vi "close.vi"(8 "error in":errorcluster, 11 "TEC runtime in":refnum<class "TEC runtime.lvclass">) -> (0 "error out":errorcluster)   [LabVIEW 2013, in "TEC runtime.lvclass"]
doc: "Provides an interface for terminating a module instance. While this interface performs no operations, a child should close and deallocate any open references or memory."
uses:
  TEC runtime.lvclass
  TEC runtime.lvclass/TEC runtime.ctl
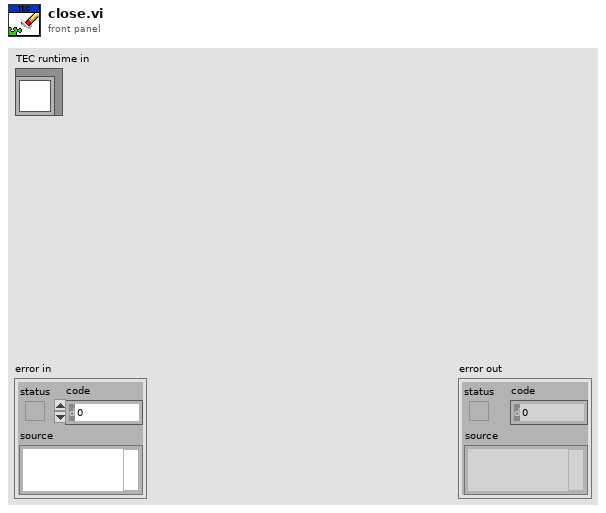
[diagram p1: front panel]
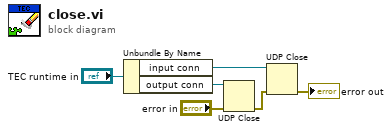
[diagram p0: block diagram]
diagram:
  n1 = Unbundle By Name("TEC runtime in") -> ("input conn"=w1:refnum<k16>, "output conn"=w2:refnum<k16>)
  n2 = UDP Close(connection ID=w2, 8:"error in") -> (error out=w4:errorcluster)  [unwired: 1 out]
  n3 = UDP Close(connection ID=w1, 8:w4) -> (error out=→"error out":errorcluster)  [unwired: 1 out]
